vi "CastSpell.vi"(8 "error in (no error)":errorcluster, 11 "MazeGame":refnum<class "MazeGame.lvclass">) -> (0 "error out":errorcluster, 2 "Spell":refnum<class "Spell.lvclass">, 3 "MazeGame":refnum<class "MazeGame.lvclass">)   [LabVIEW 2020, in "FactoryMethod.lvlib" / "ParameterizedFactoryMethod.lvlib" / "MazeGame.lvclass"]
uses:
  MazeGame.lvclass
  GoFcommonClasses/Spell/Spell.lvclass
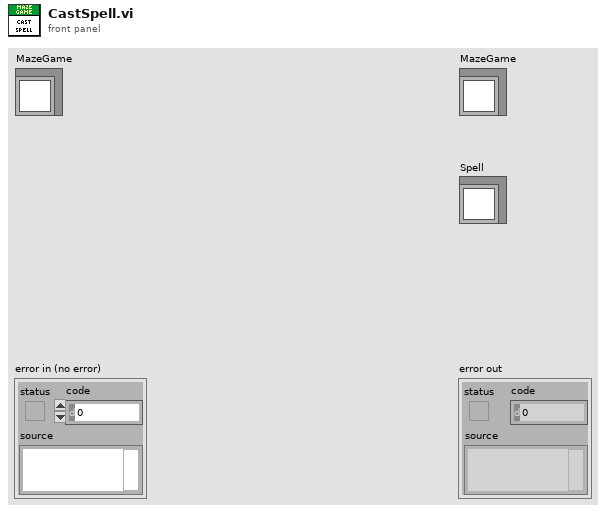
[diagram p1: front panel]
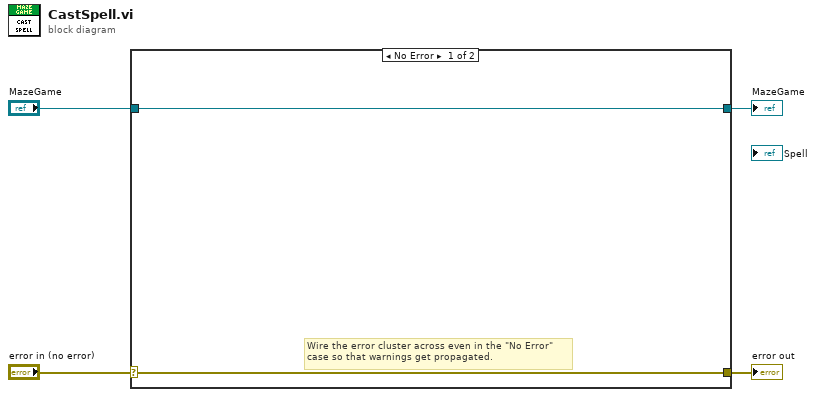
[diagram p0: block diagram]
diagram:
  n1 = case shown="No Error" "error in (no error)" {
    selector: "error in (no error)" -> [w5 w8]
    tunnel: [w5 w8] -> w3
    tunnel: [w6 w7] -> w1
    tunnel: "MazeGame" -> [w6 w7]
    frame No Error {
      # "Wire the error cluster across even in the \"No Error\"\ncase so that warnings get propagated."
    }
    frame Error {
    }
  }
  "error out" <- w3
  "MazeGame" <- w1
